vi "_RT_CtrlLoop_WfmData_Process.vi"(8 "error in (no error)":errorcluster) -> (0 "error out":errorcluster)   [LabVIEW 2018]
uses:
  PublicSubVI/Ctl/_ctl_RT_NS_Status.ctl
  PublicSubVI/Ctl/_ctl_RT_SysLog.ctl
  PublicSubVI/Ctl/_ctl_Integrated_Cmd.ctl
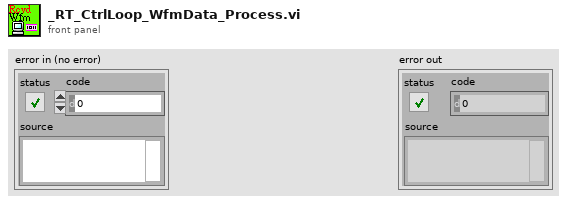
[diagram p1: front panel]
types:
  T1 = typedef "_ctl_RT_SysLog.ctl" = enum16{"None", "Initialize", "StartupRT", "StartupFPGA", "StartupAllocator", "GetMass", "SetWfmCode", "SetLaserCtrl", "SetTurboCtrl", "SetD999Ctrl", "Reconnecting...", "Interrupt", "StopRT"}
  T2 = typedef "_ctl_RT_NS_Status.ctl" = enum8{"Idle", "Init", "Connected", "Stop"}
  T3 = typedef "_ctl_Integrated_Cmd.ctl" = enum8{"Init", "Set", "Get", "Read", "Write", "Send", "Idle", "Startup", "Execution", "End", "Close"}
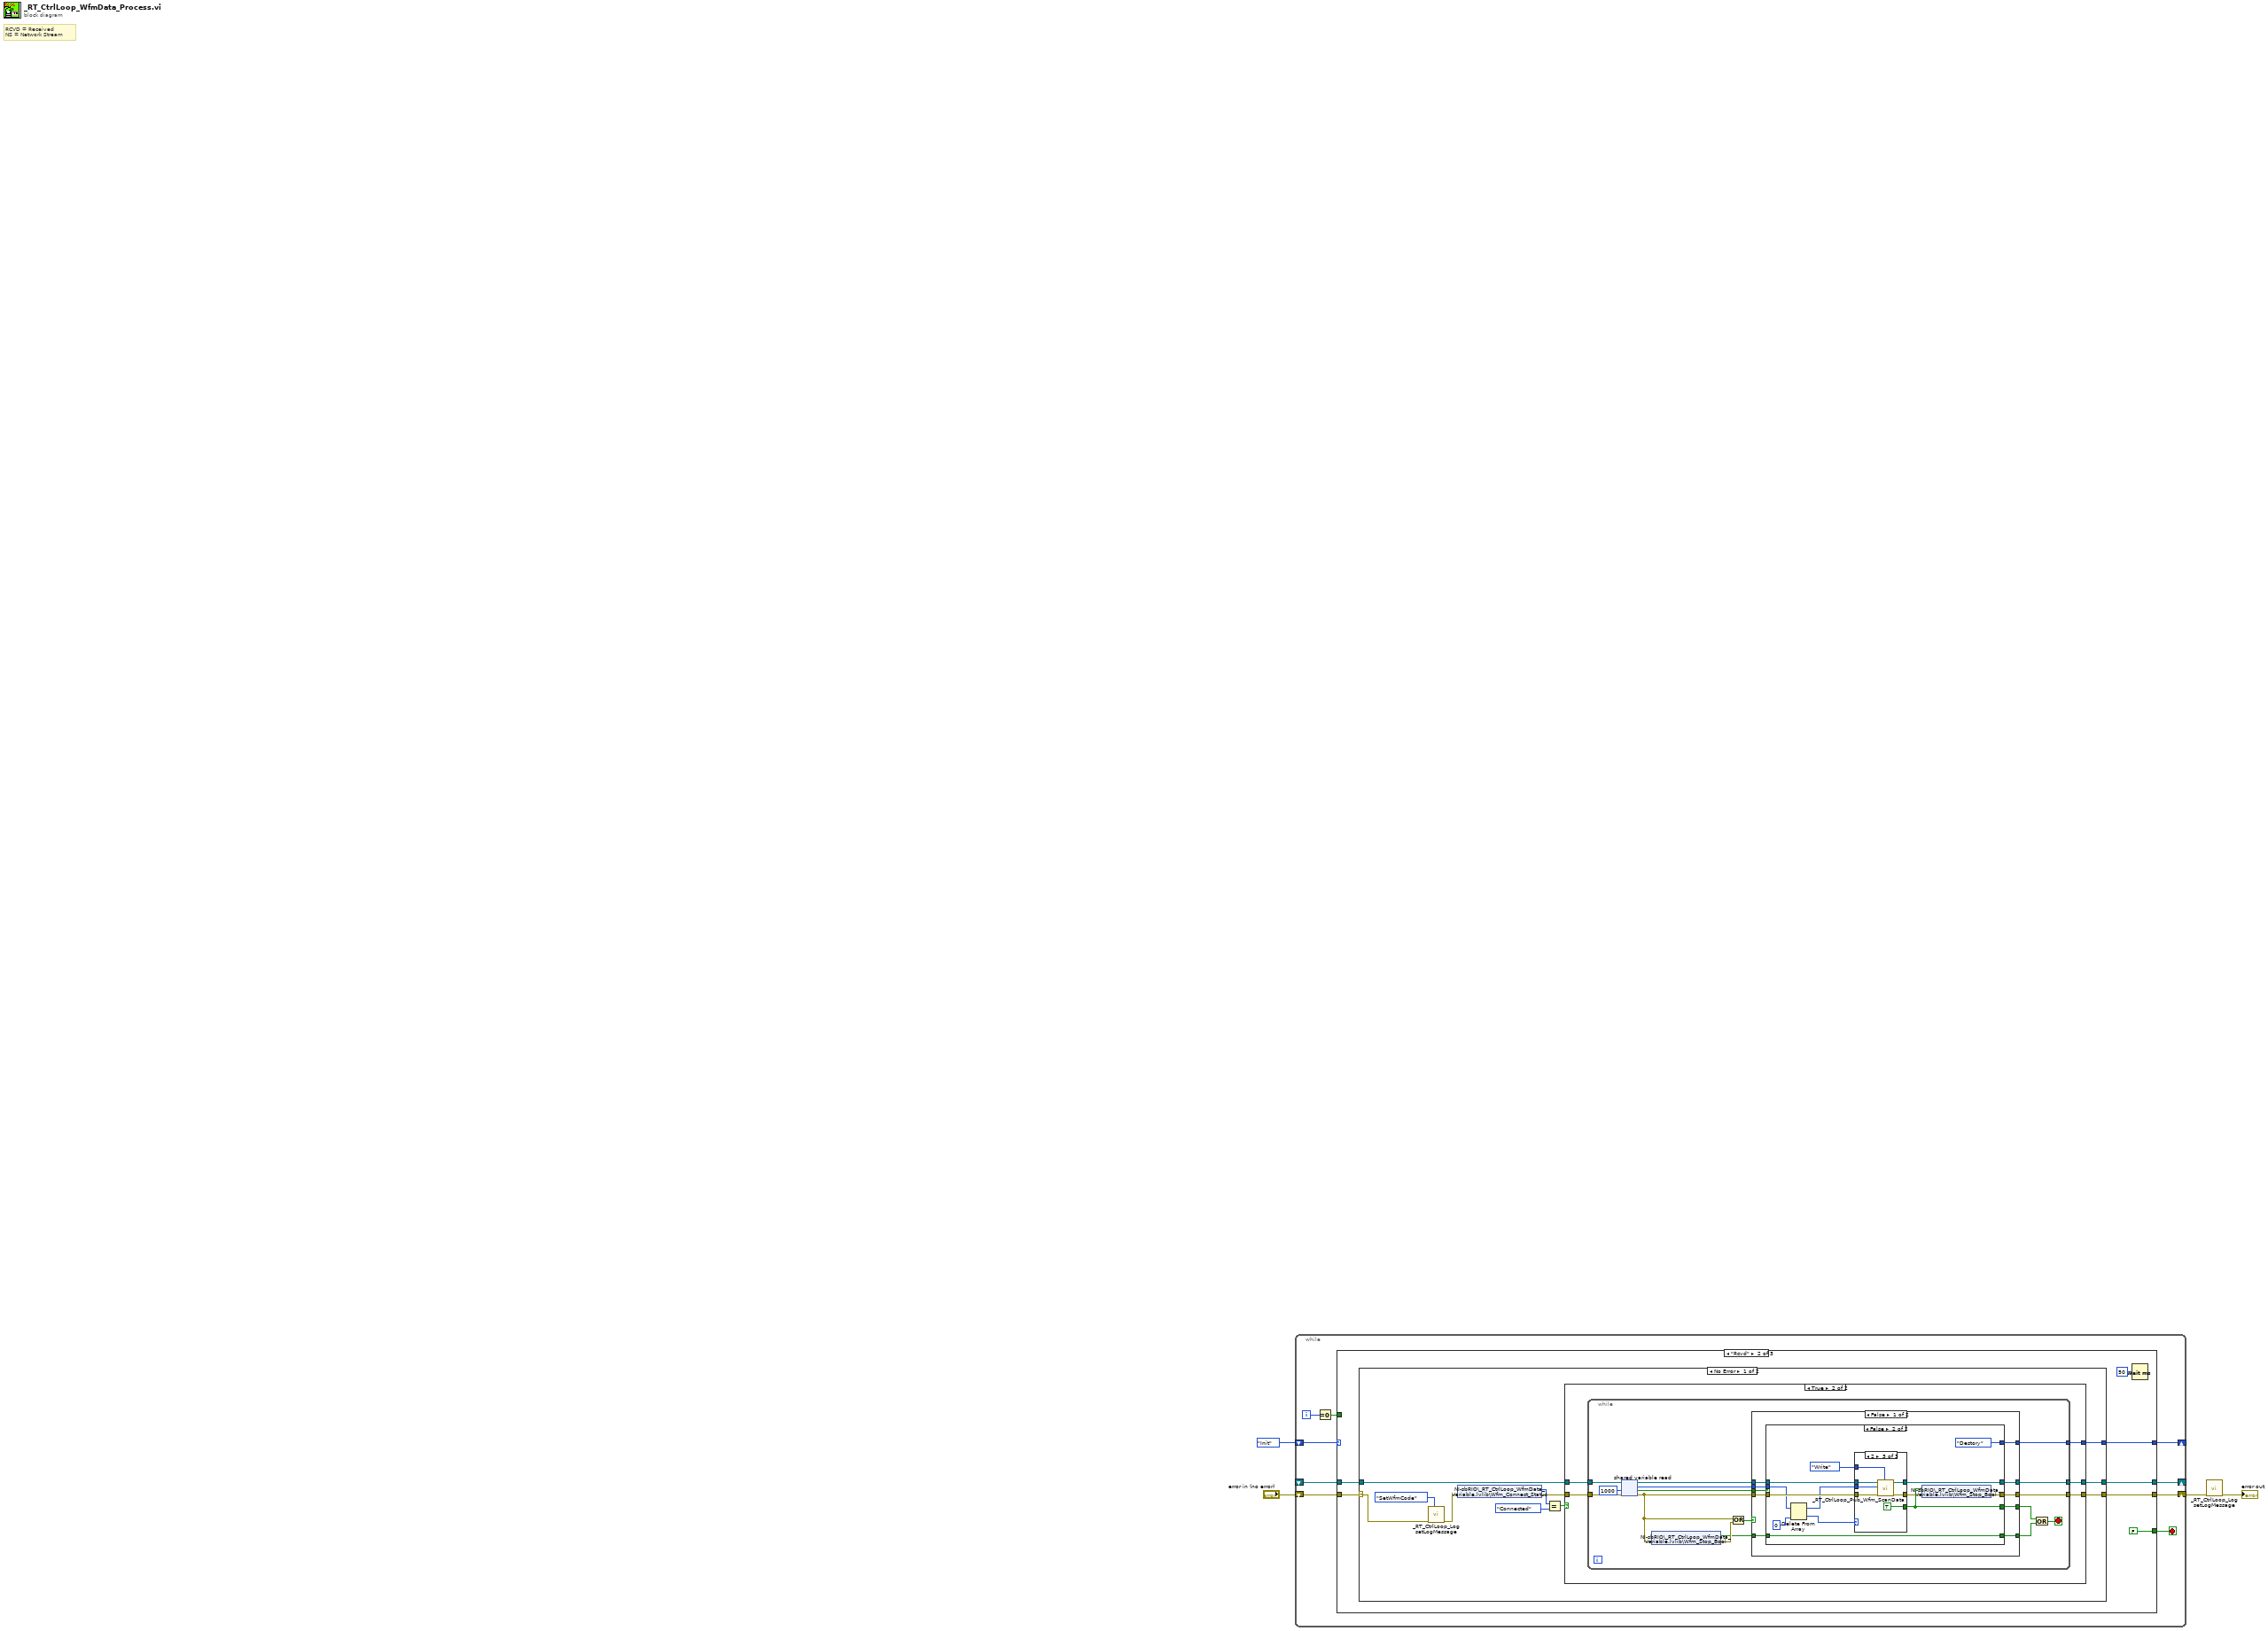
[diagram p0: block diagram]
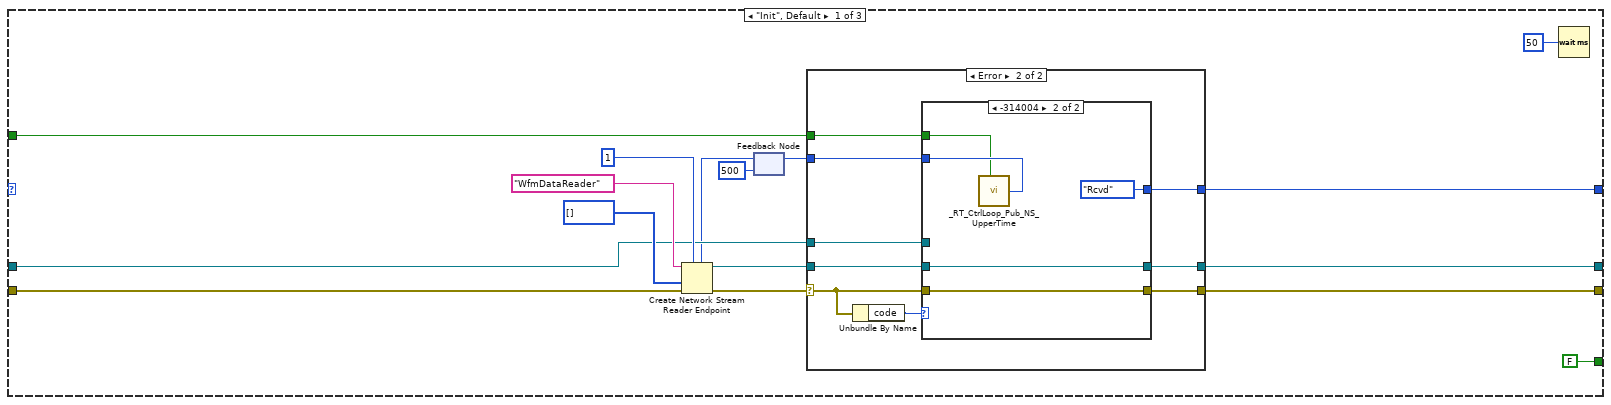
[diagram p2: hidden frame]
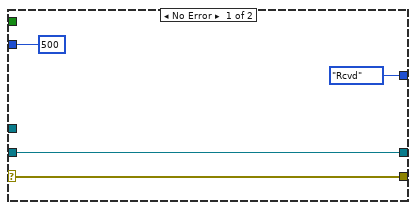
[diagram p3: hidden frame]
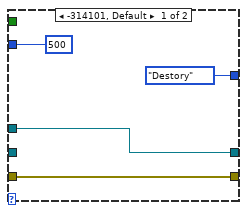
[diagram p4: hidden frame]
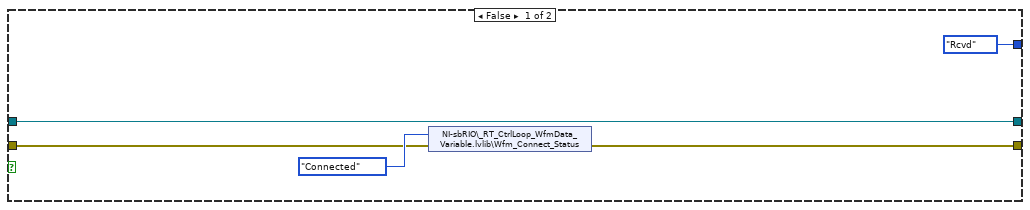
[diagram p5: hidden frame]
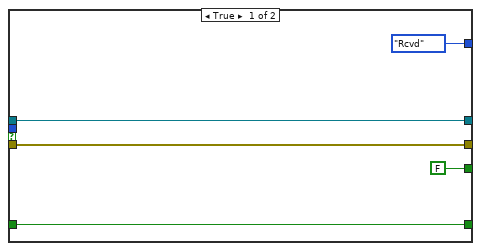
[diagram p6: hidden frame]
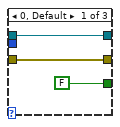
[diagram p7: hidden frame]
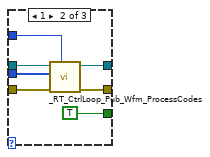
[diagram p8: hidden frame]
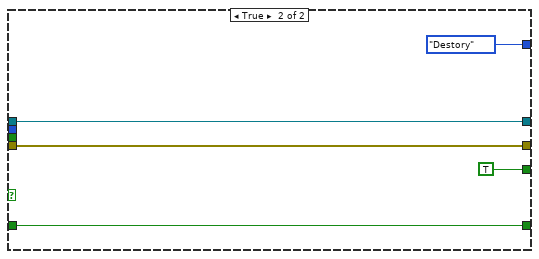
[diagram p9: hidden frame]
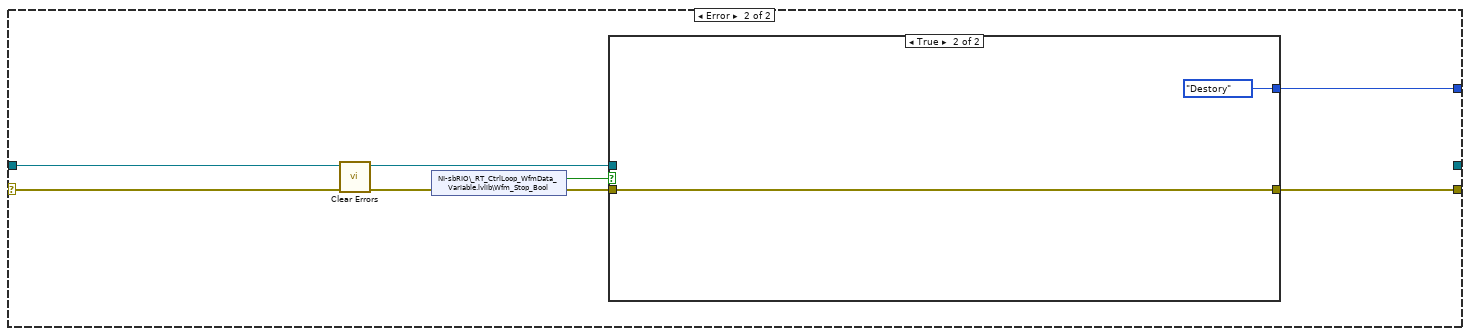
[diagram p10: hidden frame]
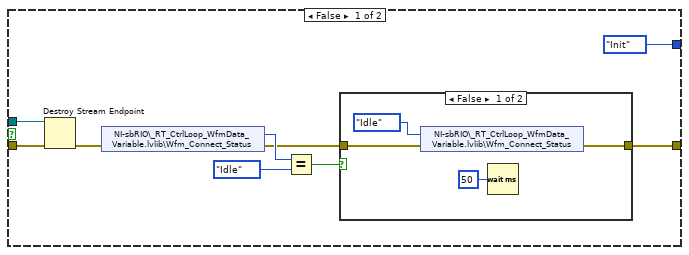
[diagram p11: hidden frame]
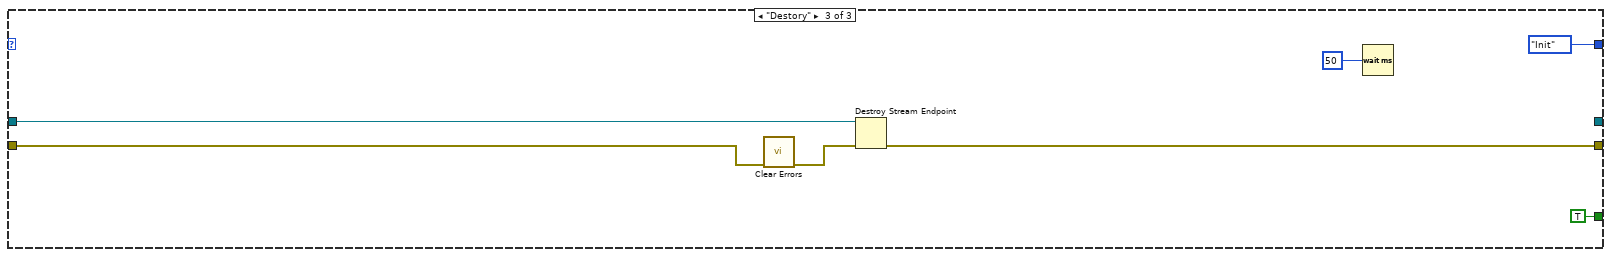
[diagram p13: hidden frame]
diagram:
  # "RCVD = Received\nNS = Network Stream"
  n1 = while {
    shift-right: [w12] -> _
    shift-left: _ -> [w11]
    shift-right: [w10] -> w2
    shift-left: "error in (no error)" -> [w9]
    shift-right: [w7] -> _
    shift-left: enum8{"Init", "Rcvd", "Destory"}."Init" -> [w8]
    i -> [w6]
    stop <- w13 stop-if-true
    n2 = Equal To 0?(x=w6) -> (x = 0?=w5:bool)
    n3 = case shown="\"Rcvd\"" w8 {
      tunnel: w9 -> [w29 w57 w172]
      tunnel: [FALSE ("Boolean") FALSE ("Boolean") TRUE ("Boolean")] -> w13
      tunnel: [w22 w53 _] -> w12
      tunnel: w11 -> [w23 w58 w171]
      tunnel: [w20 w56 w168] -> w10
      tunnel: [w21 w54 enum8{"Init", "Rcvd", "Destory"}."Init"] -> w7
      tunnel: w5 -> [w15 _ _]
      frame "Init", Default {
        n4 = feedback #1(500 ("UpdateTime")) -> (w17:i32)
        n5 = Create Network Stream Reader Endpoint(5:w17, 7:1 ("reader buffer size"), 8:w29, 9:u64[] [], 11:"WfmDataReader" ("EndPoint")) -> (0:w25:errorcluster, 3:w24:refnum<k21>)  [unwired: 2 in]
        n6 = case shown="Error" w25 {
          selector: w25 -> [w33 w40]
          tunnel: [w32 w38] -> w22
          tunnel: [w33 w41] -> w20
          tunnel: w24 -> [w32 w39]
          tunnel: w23 -> [_ w37]
          tunnel: [enum8{"Init", "Rcvd", "Destory"}."Rcvd" w36] -> w21
          tunnel: [500 ("UpdateTime") w35] -> w18
          tunnel: w15 -> [_ w34]
          frame No Error {
          }
          frame Error {
            n7 = Unbundle By Name(w40) -> ("code"=w42:i32)
            n8 = case shown="-314004" w42 {
              tunnel: [w45 w51] -> w41
              tunnel: w40 -> [w45 w51]
              tunnel: w39 -> [_ w50]
              tunnel: [w46 w50] -> w38
              tunnel: w37 -> [w46 _]
              tunnel: [enum8{"Init", "Rcvd", "Destory"}."Destory" enum8{"Init", "Rcvd", "Destory"}."Rcvd"] -> w36
              tunnel: [500 ("UpdateTime") w48] -> w35
              tunnel: w34 -> [_ w47]
              frame -314101, Default {
              }
              frame -314004 {
                n9 = call "_RT_CtrlLoop_Pub_NS_UpperTime.vi"("Init? (F)"=w47) -> ("UpdateTime"=w48:i32)  [unwired: 4 in]
              }
            }
          }
        }
        n10 = feedback-in #1(w18) -> ()
        n11 = Wait (ms)(milliseconds to wait=u32 50) -> ()  [unwired: 1 out]
      }
      frame "Rcvd" {
        n12 = case shown="No Error" w57 {
          selector: w57 -> [w61 w150]
          tunnel: w58 -> [w69 w145]
          tunnel: [w64 w149] -> w56
          tunnel: [w65 w144] -> w54
          tunnel: [w66 _] -> w53
          frame No Error {
            n13 = call "_RT_CtrlLoop_Log setLogMessage.vi"("system type"=_ctl_RT_SysLog."SetWfmCode", "error in"=w61) -> ("error out"=w60:errorcluster)  [unwired: 8 in, 1 out]
            n14 = shared-variable "NI-sbRIO\\_RT_CtrlLoop_WfmData_Variable.lvlib\\Wfm_Connect_Status"(error in=w60) -> (w68:T2, error out=w63:errorcluster)
            n15 = Equal?(x=w68, y=_ctl_RT_NS_Status."Connected") -> (x = y?=w62:bool)
            n16 = case shown="True" w62 {
              tunnel: w69 -> [w71 w79]
              tunnel: [w71 w78] -> w66
              tunnel: [enum8{"Init", "Rcvd", "Destory"}."Rcvd" w77] -> w65
              tunnel: [w72 w75] -> w64
              tunnel: w63 -> [w73 w76]
              frame False {
                n17 = shared-variable "NI-sbRIO\\_RT_CtrlLoop_WfmData_Variable.lvlib\\Wfm_Connect_Status"(_ctl_RT_NS_Status."Connected" ("Signal_RT_Status"), error in=w73) -> (error out=w72:errorcluster)
              }
              frame True {
                n18 = while {
                  tunnel: w76 -> [w94]
                  tunnel: w79 -> [w93]
                  tunnel: [w90] -> w75
                  tunnel: [w89] -> w78
                  tunnel: [w84] -> w77
                  stop <- w91 stop-if-true
                  n19 = shared-variable-read(w93, w94, 1000 ("timeout ms (-1)")) -> (w87:refnum<k21>, w83:errorcluster, w95:bool, w92:u64[])
                  n20 = shared-variable "NI-sbRIO\\_RT_CtrlLoop_WfmData_Variable.lvlib\\Wfm_Stop_Bool"(error in=w83) -> (w81:bool, error out=w82:errorcluster)
                  n21 = Or(x=w83, y=w82) -> (x .or. y?=w86:bool)
                  n22 = case shown="False" w86 {
                    tunnel: w83 -> [w103 w140]
                    tunnel: w95 -> [w105 _]
                    tunnel: w87 -> [w104 w139]
                    tunnel: [w102 w140] -> w90
                    tunnel: w92 -> [w101 _]
                    tunnel: [w100 w139] -> w89
                    tunnel: [w99 TRUE] -> w88
                    tunnel: [w98 enum8{"Init", "Rcvd", "Destory"}."Destory"] -> w84
                    tunnel: [w97 w141] -> w80
                    tunnel: w81 -> [w96 w141]
                    frame False {
                      n23 = case shown="False" w105 {
                        tunnel: w104 -> [w109 w121]
                        tunnel: w103 -> [w110 w123]
                        tunnel: [w110 w122] -> w102
                        tunnel: w101 -> [_ w115]
                        tunnel: [w109 w120] -> w100
                        tunnel: [FALSE w119] -> w99
                        tunnel: [enum8{"Init", "Rcvd", "Destory"}."Rcvd" enum8{"Init", "Rcvd", "Destory"}."Destory"] -> w98
                        tunnel: [w106 w112] -> w97
                        tunnel: w96 -> [w106 w112]
                        frame True {
                        }
                        frame False {
                          n24 = Delete From Array(array=w115, index=0) -> (deleted portion=w111:u64, array with subset deleted=w114:u64[])  [unwired: 1 in]
                          n25 = case shown="2" w111 {
                            tunnel: _ctl_Integrated_Cmd."Write" ("Enum") -> [_ w129 w133]
                            tunnel: w114 -> [_ w131 w137]
                            tunnel: [w126 w127 w134] -> w116
                            tunnel: w123 -> [w126 w130 w136]
                            tunnel: w121 -> [w125 w132 w138]
                            tunnel: [w125 w132 w138] -> w120
                            tunnel: [FALSE TRUE TRUE] -> w119
                            frame 0, Default {
                            }
                            frame 1 {
                              n26 = call "_RT_CtrlLoop_Pub_Wfm_ProcessCodes.vi"("Function"=w129, "error in (no error)"=w130, "EventCodes_U64Arr in"=w131) -> ("error out"=w127:errorcluster)  [unwired: 5 in, 3 out]
                            }
                            frame 2 {
                              n27 = call "_RT_CtrlLoop_Pub_Wfm_ScanData.vi"("Function"=w133, "error in (no error)"=w136, "WFM_U64Arr in"=w137) -> ("error out"=w134:errorcluster)  [unwired: 7 in, 1 out]
                            }
                          }
                          n28 = shared-variable "NI-sbRIO\\_RT_CtrlLoop_WfmData_Variable.lvlib\\Wfm_Stop_Bool"(w119, error in=w116) -> (error out=w122:errorcluster)
                        }
                      }
                    }
                    frame True {
                    }
                  }
                  n29 = Or(x=w88, y=w80) -> (x .or. y?=w91:bool)
                }
              }
            }
          }
          frame Error {
            n30 = call <vilib>:"Clear Errors.vi"("error in (no error)"=w150) -> ("error out"=w148:errorcluster)  [unwired: 5 in, 1 out]
            n31 = shared-variable "NI-sbRIO\\_RT_CtrlLoop_WfmData_Variable.lvlib\\Wfm_Stop_Bool"(error in=w148) -> (w146:bool, error out=w147:errorcluster)
            n32 = case shown="True" w146 {
              tunnel: w147 -> [w156 w166]
              tunnel: w145 -> [w154 _]
              tunnel: [w152 w166] -> w149
              tunnel: [enum8{"Init", "Rcvd", "Destory"}."Init" enum8{"Init", "Rcvd", "Destory"}."Destory"] -> w144
              frame False {
                n33 = Destroy Stream Endpoint(8:w156, 11:w154) -> (0:w155:errorcluster)
                n34 = shared-variable "NI-sbRIO\\_RT_CtrlLoop_WfmData_Variable.lvlib\\Wfm_Connect_Status"(error in=w155) -> (w157:T2, error out=w153:errorcluster)
                n35 = Equal?(x=w157, y=_ctl_RT_NS_Status."Idle") -> (x = y?=w159:bool)
                n36 = case shown="False" w159 {
                  tunnel: w153 -> [w162 w164]
                  tunnel: [w163 w164] -> w152
                  frame False {
                    n37 = shared-variable "NI-sbRIO\\_RT_CtrlLoop_WfmData_Variable.lvlib\\Wfm_Connect_Status"(_ctl_RT_NS_Status."Idle" ("Signal_RT_Status"), error in=w162) -> (error out=w163:errorcluster)
                    n38 = Wait (ms)(milliseconds to wait=u32 50) -> ()  [unwired: 1 out]
                  }
                  frame True {
                  }
                }
              }
              frame True {
              }
            }
          }
        }
        n39 = Wait (ms)(milliseconds to wait=u32 50) -> ()  [unwired: 1 out]
      }
      frame "Destory" {
        n40 = call <vilib>:"Clear Errors.vi"("error in (no error)"=w172) -> ("error out"=w173:errorcluster)  [unwired: 5 in, 1 out]
        n41 = Destroy Stream Endpoint(8:w173, 11:w171) -> (0:w168:errorcluster)
        n42 = Wait (ms)(milliseconds to wait=u32 50) -> ()  [unwired: 1 out]
      }
    }
  }
  n43 = call "_RT_CtrlLoop_Log setLogMessage.vi"("error in"=w2) -> ("error out"=→"error out":errorcluster)  [unwired: 9 in, 1 out]
